vi "Close Cmd Connection.vi"(8 "error in (no error)":errorcluster, 11 "FTP in":refnum<class "FTP.lvclass">) -> (0 "error out":errorcluster, 3 "FTP out":refnum<class "FTP.lvclass">)   [LabVIEW 2020, in "FTP.lvlib" / "FTP.lvclass"]
uses:
  FTP.lvclass
  FTP.lvclass/FTP.ctl
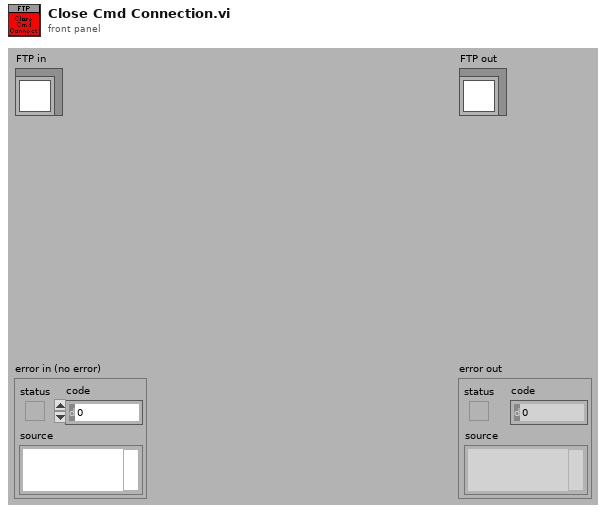
[diagram p1: front panel]
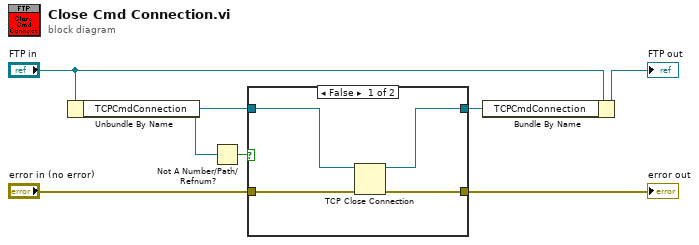
[diagram p0: block diagram]
diagram:
  n1 = Unbundle By Name("FTP in") -> ("TCPCmdConnection"=w1:refnum<k5>)
  n2 = Not A Number/Path/Refnum?(number/path/refnum=w1) -> (NaN/Path/Refnum?=w2:bool)
  n3 = case shown="False" w2 {
    tunnel: [w11 w12] -> w7
    tunnel: w1 -> [w10 w13]
    tunnel: [w9 w13] -> w4
    tunnel: "error in (no error)" -> [w8 w12]
    frame False {
      n4 = TCP Close Connection(connection ID=w10, error in (no error)=w8) -> (connection ID out=w9:refnum<k5>, error out=w11:errorcluster)  [unwired: 1 in]
    }
    frame True {
    }
  }
  "error out" <- w7
  n5 = Bundle By Name(cluster="FTP in", "TCPCmdConnection"=w4) -> (→"FTP out":refnum<class "FTP.lvclass">)
